vi "C4Buf_readFeature.vi"(0 "c4buf in":refnum<k24>, 5 "name in":string, 11 "error in":errorcluster) -> (4 "c4buf out":refnum<k24>, 6 "value out":string, 15 "error out":errorcluster)   [LabVIEW 2015, in "libC4HdlLV.lvlib"]
uses:
  libC4HdlLV.lvlib
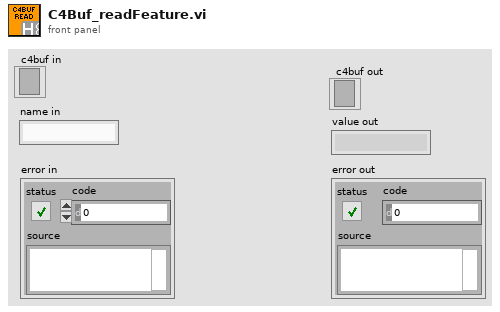
[diagram p1: front panel]
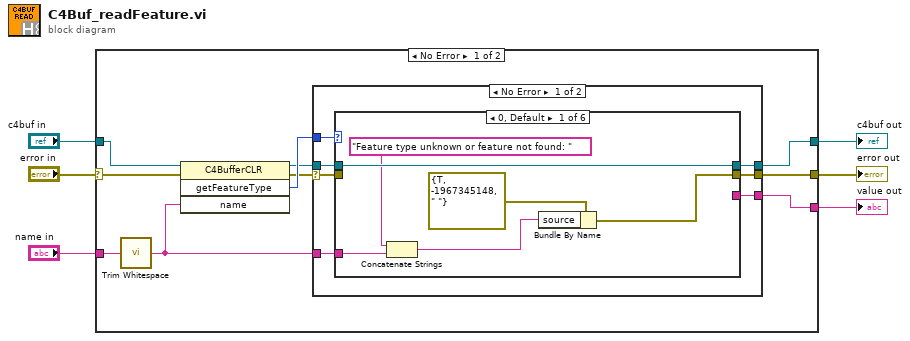
[diagram p0: block diagram]
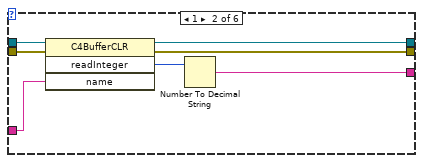
[diagram p2: hidden frame]
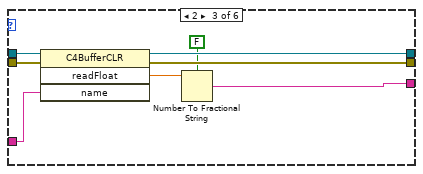
[diagram p3: hidden frame]
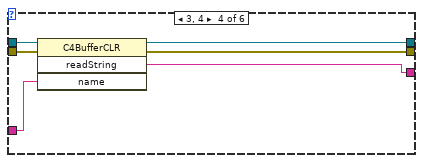
[diagram p4: hidden frame]
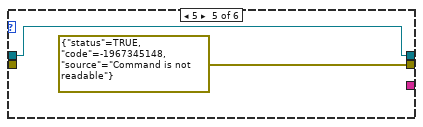
[diagram p5: hidden frame]
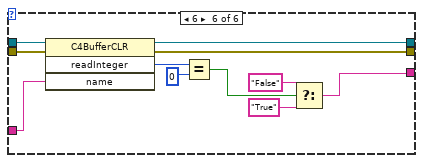
[diagram p6: hidden frame]
diagram:
  n1 = case shown="No Error" "error in" {
    selector: "error in" -> [w12 w67]
    tunnel: [w16 w66] -> w1
    tunnel: [w15 w67] -> w4
    tunnel: "name in" -> [w14 _]
    tunnel: "c4buf in" -> [w11 w66]
    tunnel: [w13 _] -> w5
    frame No Error {
      n2 = call <vilib>:"Trim Whitespace.vi"("string"=w14) -> ("trimmed string"=w10:string)  [unwired: 1 in]
      n3 = invoke class="C4BufferCLR" method="getFeatureType"(reference=w11, error in=w12, "name"=w10) -> (reference out=w8:refnum<k24>, error out=w7:errorcluster, "getFeatureType"=w9:i64)  [unwired: 1 in, 1 out]
      n4 = case shown="No Error" w7 {
        selector: w7 -> [w17 w65]
        tunnel: [w23 w64] -> w16
        tunnel: [w22 w65] -> w15
        tunnel: [w21 _] -> w13
        tunnel: w10 -> [w20 _]
        tunnel: w9 -> [w19 _]
        tunnel: w8 -> [w18 w64]
        frame No Error {
          n5 = case shown="0, Default" w19 {
            tunnel: w18 -> [w29 w36 w37 w50 w52 w63]
            tunnel: w17 -> [_ w35 w44 w49 _ w62]
            tunnel: w20 -> [w24 w34 w43 w48 _ w61]
            tunnel: [w29 w33 w42 w47 w52 w60] -> w23
            tunnel: [w26 w32 w41 w46 errorcluster {"status"=TRUE, "code"=-1967345148, "source"="Command is not readable"} ("error out") w59] -> w22
            tunnel: [_ w30 w39 w45 _ w53] -> w21
            frame 0, Default {
              n6 = Concatenate Strings("Feature type unknown or feature not found: " ("source"), w24) -> (w27:string)
              n7 = Bundle By Name(cluster=errorcluster {"status"=TRUE, "code"=-1967345148, "source"=" "} ("error out"), "source"=w27) -> (w26:errorcluster)
            }
            frame 1 {
              n8 = invoke class="C4BufferCLR" method="readInteger"(reference=w36, error in=w35, "name"=w34) -> (reference out=w33:refnum<k24>, error out=w32:errorcluster, "readInteger"=w31:i64)  [unwired: 1 in, 1 out]
              n9 = Number To Decimal String(number=w31) -> (decimal integer string=w30:string)  [unwired: 1 in]
            }
            frame 2 {
              n10 = invoke class="C4BufferCLR" method="readFloat"(reference=w37, error in=w44, "name"=w43) -> (reference out=w42:refnum<k24>, error out=w41:errorcluster, "readFloat"=w40:dbl)  [unwired: 1 in, 1 out]
              n11 = Number To Fractional String(use system decimal point (T)=FALSE, number=w40) -> (F-format string=w39:string)  [unwired: 2 in]
            }
            frame 3, 4 {
              n12 = invoke class="C4BufferCLR" method="readString"(reference=w50, error in=w49, "name"=w48) -> (reference out=w47:refnum<k24>, error out=w46:errorcluster, "readString"=w45:string)  [unwired: 1 in, 1 out]
            }
            frame 5 {
            }
            frame 6 {
              n13 = invoke class="C4BufferCLR" method="readInteger"(reference=w63, error in=w62, "name"=w61) -> (reference out=w60:refnum<k24>, error out=w59:errorcluster, "readInteger"=w58:i64)  [unwired: 1 in, 1 out]
              n14 = Equal?(x=w58, y=i64 0) -> (x = y?=w56:bool)
              n15 = Select(t="False", s=w56, f="True") -> (s? t:f=w53:string)
            }
          }
        }
        frame Error {
        }
      }
    }
    frame Error {
    }
  }
  "value out" <- w5
  "error out" <- w4
  "c4buf out" <- w1
